vi "xml test.vi"() -> ()   [LabVIEW 2015]
panel:
  out "值 2":dbl
  in  "xml字符串 2":string
  out "值":cluster{"值":dbl, "布尔":bool}
  in  "簇":cluster{"值":dbl, "布尔":bool}
  out "xml字符串":string
  in  "数值":dbl
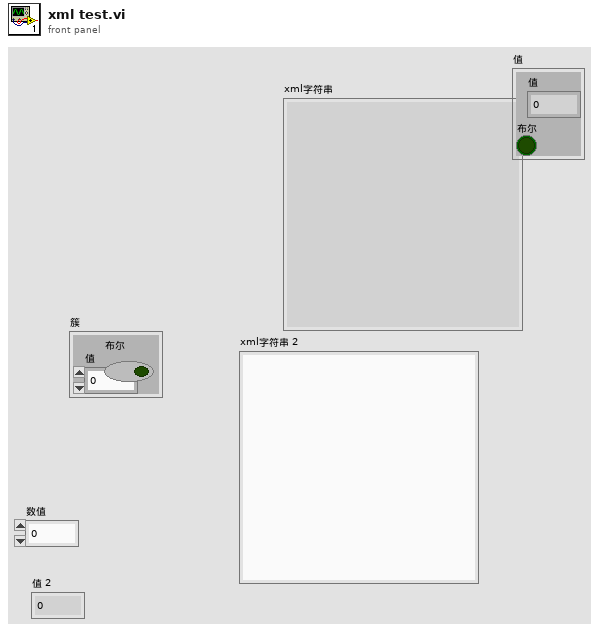
[diagram p1: front panel]
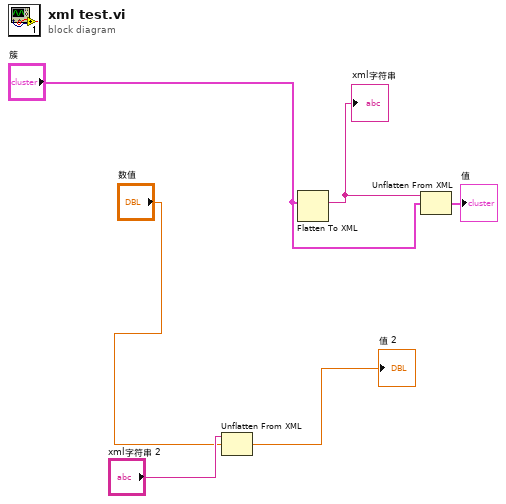
[diagram p0: block diagram]
diagram:
  n1 = Unflatten From XML(xml string="xml字符串 2", type="数值") -> (value=→"值 2":dbl)  [unwired: 1 in, 1 out]
  n2 = Flatten To XML(anything="簇") -> (xml string=w5:string)
  "xml字符串" <- w5
  n3 = Unflatten From XML(xml string=w5, type="簇") -> (value=→"值":cluster{"值":dbl, "布尔":bool})  [unwired: 1 in, 1 out]
